vi "getConnectionPoints.vi"(0 "reference":refnum<class "NoteEdge.lvclass">, 5 "error in (no error)":errorcluster) -> (14 "reference out":refnum<class "NoteEdge.lvclass">, 15 "connectionPoints":T1[](array[typedef]) {"y" format="%.2f"; "x" format="%.2f"}, 19 "error out":errorcluster)   [LabVIEW 2016, in "NoteEdge.lvclass"]
doc: "public Line2D getConnectionPoints()"
uses:
  <resource>/Framework/Providers/Open_GDS/UML/NoteEdge_class/NoteEdge.lvclass
  C:/Program Files (x86)/National Instruments/LabVIEW 2016/resource/Framework/Providers/Open_GDS/UML/AbstractEdge_class/AbstractEdge.lvclass
  <resource>/Framework/Providers/Open_GDS/UML/General/Point/Point Point2D.ctl
  <resource>/Framework/Providers/Open_GDS/UML/AbstractNode_class/AbstractNode.lvclass
  <resource>/Framework/Providers/Open_GDS/UML/Direction_class/Direction.lvclass
  <resource>/Framework/Providers/Open_GDS/UML/AbstractEdge_class/AbstractEdge.lvclass
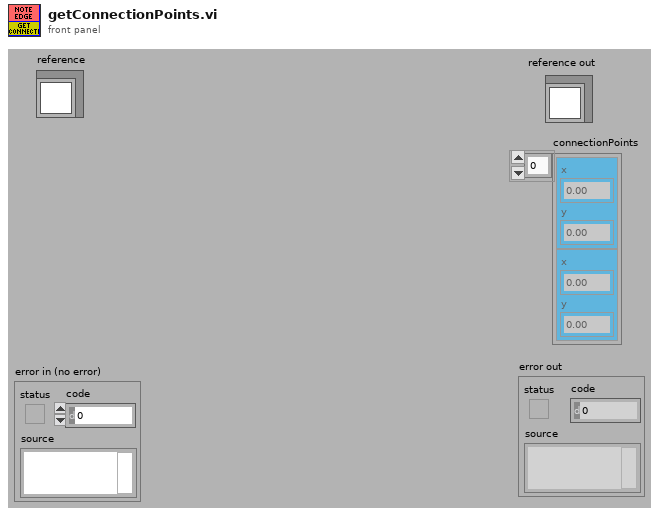
[diagram p1: front panel]
types:
  T1 = typedef "Point Point2D.ctl" = cluster{"x":dbl, "y":dbl}
  T2 = typedef "AbstractEdge.lvclass/ObjectAttributes.ctl" = cluster{"start":refnum<class "AbstractNode.lvclass">, "end":refnum<class "AbstractNode.lvclass">}
  T3 = typedef "Rectangle Rectangle2D.ctl" = cluster{"x":dbl, "y":dbl, "width":dbl, "height":dbl}
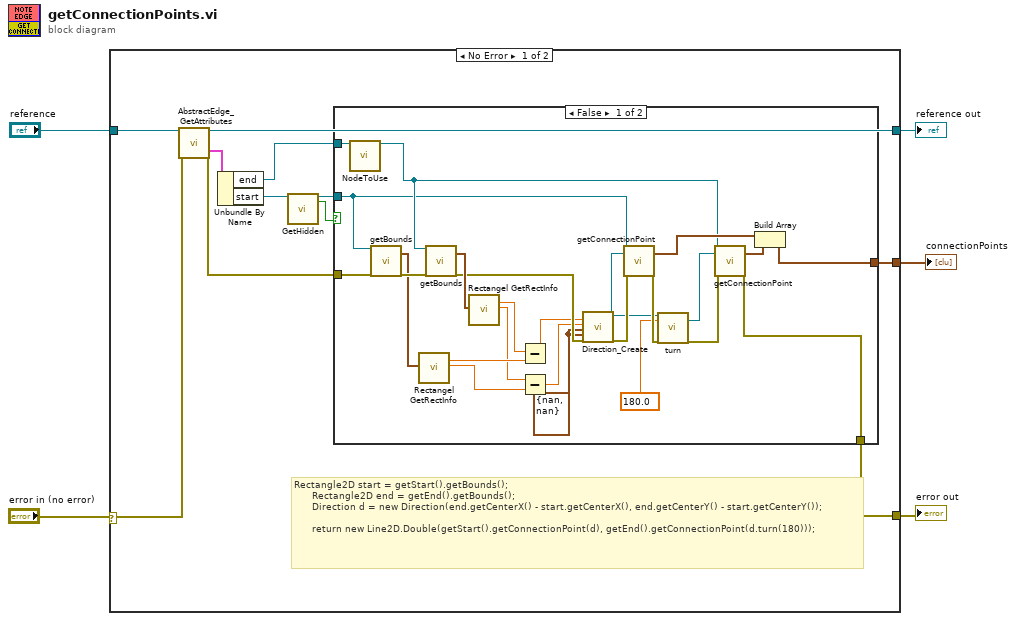
[diagram p0: block diagram]
diagram:
  n1 = case shown="No Error" "error in (no error)" {
    selector: "error in (no error)" -> [w11 w43]
    tunnel: "reference" -> [w16 w44]
    tunnel: [w15 w43] -> w4
    tunnel: [w14 w44] -> w3
    tunnel: [w13 _] -> w1
    frame No Error {
      # "Rectangle2D start = getStart().getBounds();\n      Rectangle2D end = getEnd().getBounds();\n      Direction d = new Direction(end.getCenterX() - start.getCenterX(), end.getCenterY() - start.getCenterY());\n\n      return new Line2D.Double(getStart().getConnectionPoint(d), getEnd().getConnectionPoint(d.turn(180)));"
      n2 = call <resource>:"AbstractEdge_GetAttributes.vi"("reference in"=w16, "error in (no error)"=w11) -> ("reference out"=w14:refnum<class "NoteEdge.lvclass">, "Data"=w6:T2, "error out"=w12:errorcluster)  [unwired: 14 in, 1 out]
      n3 = Unbundle By Name(w6) -> ("end"=w10:refnum<class "AbstractNode.lvclass">, "start"=w9:refnum<class "AbstractNode.lvclass">)
      n4 = call-dynamic "GetHidden.vi"("reference in"=w9) -> ("reference out"=w8:refnum<class "AbstractNode.lvclass">, "Hidden"=w7:bool)  [unwired: 16 in, 1 out]
      n5 = case shown="False" w7 {
        tunnel: [w17 w42] -> w15
        tunnel: [w41 _] -> w13
        tunnel: w12 -> [w28 w42]
        tunnel: w10 -> [w21 _]
        tunnel: w8 -> [w19 _]
        frame False {
          w18 = T1 {"x"=nan, "y"=nan} ("p1")
          n6 = call <resource>:"NodeToUse.vi"("reference in"=w21) -> ("reference out"=w20:refnum<class "AbstractNode.lvclass">)  [unwired: 15 in, 3 out]
          n7 = call-dynamic "getBounds.vi"("reference"=w19, "error in (no error)"=w28) -> ("bounds"=w39:T3, "error out"=w40:errorcluster)  [unwired: 15 in, 1 out]
          n8 = call <resource>:"Rectangel GetRectInfo.vi"("bounds"=w39) -> ("centerX"=w26:dbl, "centerY"=w24:dbl)  [unwired: 1 in, 16 out]
          n9 = call-dynamic "getBounds.vi"("reference"=w20, "error in (no error)"=w40) -> ("bounds"=w38:T3, "error out"=w37:errorcluster)  [unwired: 15 in, 1 out]
          n10 = call <resource>:"Rectangel GetRectInfo.vi"("bounds"=w38) -> ("centerX"=w27:dbl, "centerY"=w25:dbl)  [unwired: 1 in, 16 out]
          n11 = Subtract(x=w27, y=w26) -> (x-y=w23:dbl)
          n12 = Subtract(x=w25, y=w24) -> (x-y=w22:dbl)
          n13 = call <resource>:"Direction_Create.vi"("dx"=w23, "dy"=w22, "p1"=w18, "p2"=w18, "error in (no error)"=w37) -> ("reference out"=w31:refnum<class "Direction.lvclass">, "error out"=w34:errorcluster)  [unwired: 13 in]
          n14 = call-dynamic "getConnectionPoint.vi"("reference"=w19, "direction"=w31, "error in (no error)"=w34) -> ("point2D"=w36:T1, "error out"=w32:errorcluster)  [unwired: 14 in, 1 out]
          n15 = call <resource>:"turn.vi"("reference"=w31, "angle"=180.0 ("degrees"), "error in (no error)"=w32) -> ("turnedDirection"=w29:refnum<class "Direction.lvclass">, "error out"=w33:errorcluster)  [unwired: 15 out]
          n16 = call-dynamic "getConnectionPoint.vi"("reference"=w20, "direction"=w29, "error in (no error)"=w33) -> ("point2D"=w35:T1, "error out"=w17:errorcluster)  [unwired: 14 in, 1 out]
          n17 = Build Array(w36, w35) -> (w41:T1[])
        }
        frame True {
        }
      }
    }
    frame Error {
    }
  }
  "reference out" <- w3
  "error out" <- w4
  "connectionPoints" <- w1
